vi "Convert Strings to Results.vi"(8 "error in (no error)":errorcluster, 10 "path":path=path "C:/Users/Shivam/Desktop/test max.txt", 11 "Gas":string) -> (0 "error out":errorcluster, 3 "Results":T1[](array[typedef]))   [LabVIEW 2015]
uses:
  Controls/Test Info.ctl
  Controls/Total Gases.ctl
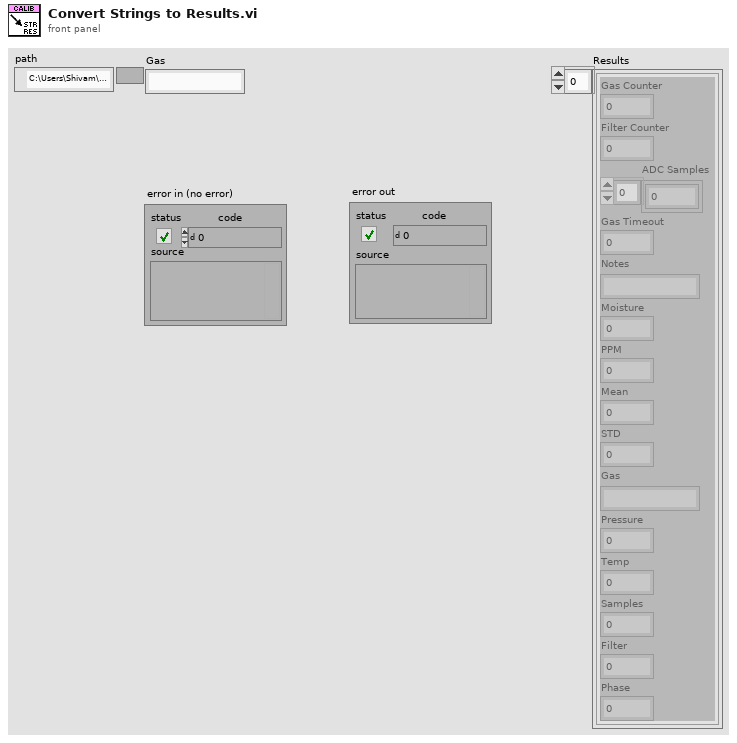
[diagram p1: front panel]
types:
  T1 = typedef "Test Info.ctl" = cluster{"Gas Counter":u16, "Filter Counter":u16, "ADC Samples":dbl[], "Gas Timeout":u16, "Notes":string, "Moisture":dbl, "PPM":dbl, "Mean":dbl, "STD":dbl, "Gas":string, "Pressure":dbl, "Temp":dbl, "Samples":u16, "Filter":u8, "Phase":dbl}
  T2 = typedef "Total Gases.ctl" = enum16{"N2", "CH4", "C2H6", "C2H4", "C2H2", "CO", "CO2", "H2O", "O2", "H2", "C3H8", "C3H6"}
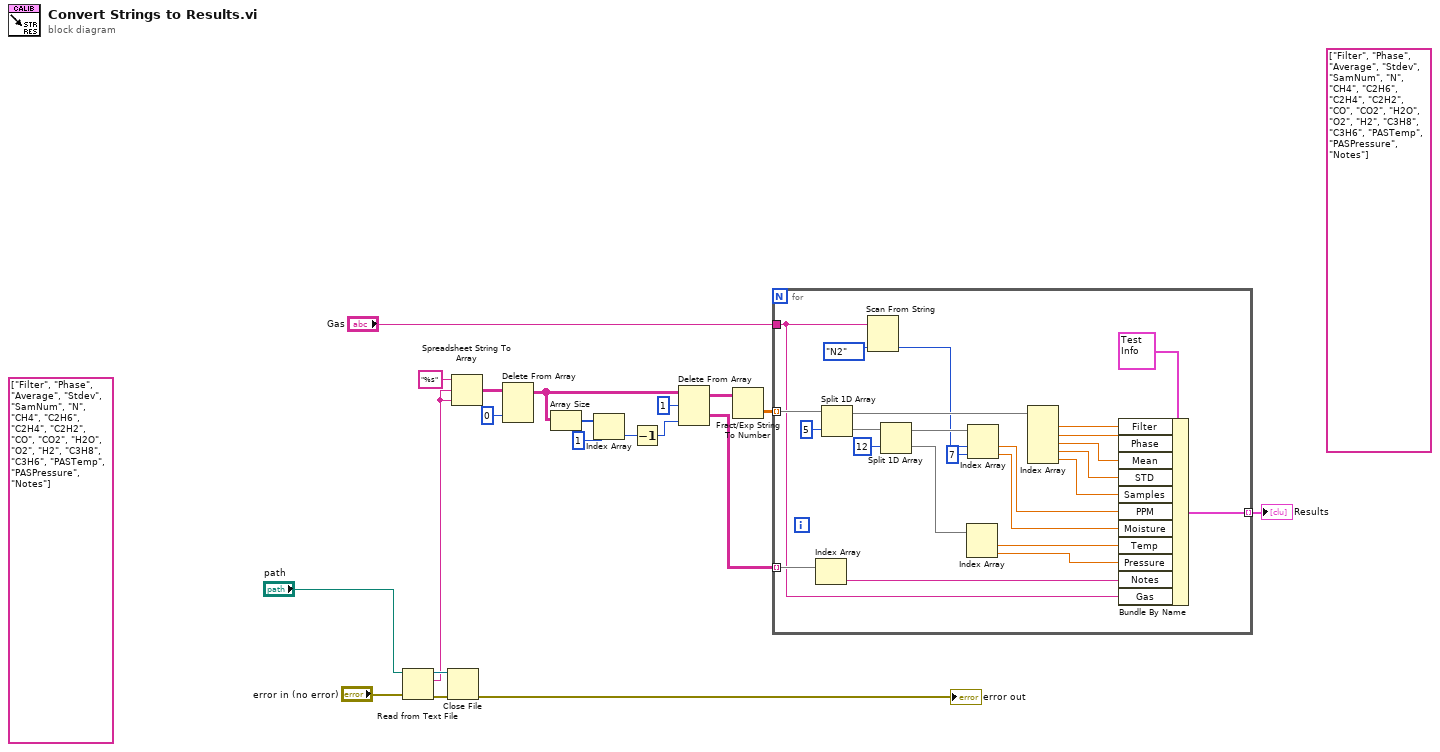
[diagram p0: block diagram]
diagram:
  (unwired) string[] ["Filter", "Phase", "Average", "Stdev", "SamNum", "N", "CH4", "C2H6", "C2H4", "C2H2", "CO", "CO2", "H2O", "O2", "H2", "C3H8", "C3H6", "PASTemp", "PASPressure", "Notes"]
  (unwired) string[] ["Filter", "Phase", "Average", "Stdev", "SamNum", "N", "CH4", "C2H6", "C2H4", "C2H2", "CO", "CO2", "H2O", "O2", "H2", "C3H8", "C3H6", "PASTemp", "PASPressure", "Notes"]
  n1 = Read from Text File(file (use dialog)="path", error in="error in (no error)") -> (refnum out=w18:refnum<file>, text=w17:string, error out=w19:errorcluster)  [unwired: 2 in, 1 out]
  n2 = Close File(refnum=w18, error in=w19) -> (error out=→"error out":errorcluster)  [unwired: 1 out]
  n3 = Spreadsheet String To Array(format string="%s", spreadsheet string=w17, array type (2D Dbl)=w17) -> (array=w15:string[][])  [unwired: 1 in]
  n4 = Delete From Array(array=w15, index (row)=0) -> (array with subset deleted=w11:string[][])  [unwired: 2 in, 1 out]
  n5 = Array Size(array=w11) -> (size(s)=w10:i32[])
  n6 = Index Array(array=w10, index=1) -> (element=w9:i32)
  n7 = Decrement(x=w9) -> (x-1=w8:i32)
  n8 = Delete From Array(array=w11, length=1, index (col)=w8) -> (deleted portion=w5:string[][], array with subset deleted=w6:string[][])  [unwired: 1 in]
  n9 = Fract/Exp String To Number(string=w6) -> (number=w13:dbl[][])  [unwired: 3 in, 1 out]
  n10 = for {
    tunnel: w13 -> [w37] mode=indexing
    tunnel: "Gas" -> [w21]
    tunnel: w5 -> [w24] mode=indexing
    tunnel: [w22] -> w4 mode=indexing
    n11 = Index Array(array=w24) -> (element=w23:string)  [unwired: 1 in]
    n12 = Split 1D Array(array=w37, index=5) -> (first subarray=w35:dbl[], second subarray=w34:dbl[])
    n13 = Scan From String(input string=w21, default 1=Total_Gases."N2" ("Gases")) -> (output 1=w31:T2)  [unwired: 3 in, 3 out]
    n14 = Split 1D Array(array=w34, index=12) -> (first subarray=w32:dbl[], second subarray=w27:dbl[])
    n15 = Index Array(array=w27) -> (element #1=w26:dbl, element #2=w25:dbl)  [unwired: 2 in]
    n16 = Index Array(array=w32, index #1=w31, index #2=7 ("index")) -> (element #1=w30:dbl, element #2=w28:dbl)
    n17 = Index Array(array=w35) -> (element #1=w43:dbl, element #2=w42:dbl, element #3=w41:dbl, element #4=w40:dbl, element #5=w39:dbl)  [unwired: 5 in]
    n18 = Bundle By Name(cluster=T1 {"Gas Counter"=0, "Filter Counter"=0, "ADC Samples"=[], "Gas Timeout"=0, "Notes"="", "Moisture"=0.0, "PPM"=0.0, "Mean"=0.0, "STD"=0.0, "Gas"="", "Pressure"=0.0, "Temp"=0.0, "Samples"=0, "Filter"=0, "Phase"=0.0} ("Test Info"), "Filter"=w43, "Phase"=w42, "Mean"=w41, "STD"=w40, "Samples"=w39, "PPM"=w30, "Moisture"=w28, "Temp"=w26, "Pressure"=w25, "Notes"=w23, "Gas"=w21) -> (w22:T1)
  }
  "Results" <- w4
